vi "Generator_sygnalu_modulujacego.vi"(10 "Parametry_cosinusow":T1, 11 "Czas":dbl) -> (3 "Sygnal_modulujacy":dbl)   [LabVIEW 2020]
doc: "VI zwraca wartosci sygnalu modulujacego stanowiacego sume sygnalow sinusoidalnych"
uses:
  Kontrolki/Parametry_cosinusow.ctl
  Kontrolki/Parametry_cosinusa.ctl
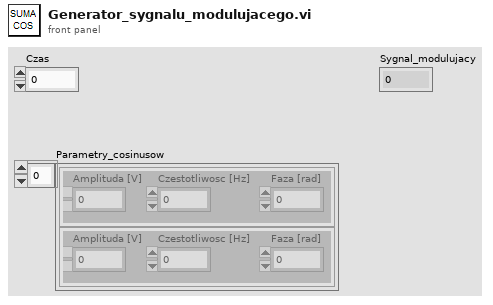
[diagram p1: front panel]
types:
  T1 = typedef "Parametry_cosinusow.ctl" = T2[]
  T2 = typedef "Parametry_cosinusa.ctl" = cluster{"Amplituda [V]":dbl, "Czestotliwosc [Hz] ":dbl, "Faza [rad]":dbl}
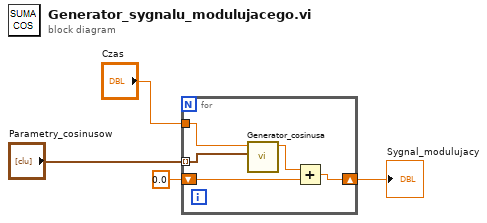
[diagram p0: block diagram]
diagram:
  n1 = for {
    tunnel: "Parametry_cosinusow" -> [w9] mode=indexing
    tunnel: "Czas" -> [w8]
    shift-right: [w5] -> w3
    shift-left: 0.0 -> [w6]
    n2 = call "Generator_cosinusa.vi"("Parametry_cosinusa"=w9, "Czas"=w8) -> ("A cos(2pift + phi)"=w7:dbl)  [unwired: 9 in]
    n3 = Add(x=w7, y=w6) -> (x+y=w5:dbl)
  }
  "Sygnal_modulujacy" <- w3
